vi "cipher data.vi"(8 "error in":errorcluster, 10 "data in":string, 11 "lvlibcrypto digest in":refnum<class "lvlibcrypto cipher.lvclass">) -> (0 "error out":errorcluster, 2 "data out":string, 3 "lvlibcrypto digest out":refnum<class "lvlibcrypto cipher.lvclass">)   [LabVIEW 2016, in "lvlibcrypto cipher.lvclass"]
uses:
  lvlibcrypto cipher.lvclass
  lvlibcrypto cipher.lvclass/lvlibcrypto cipher.ctl
  lv tls dll.lvlib
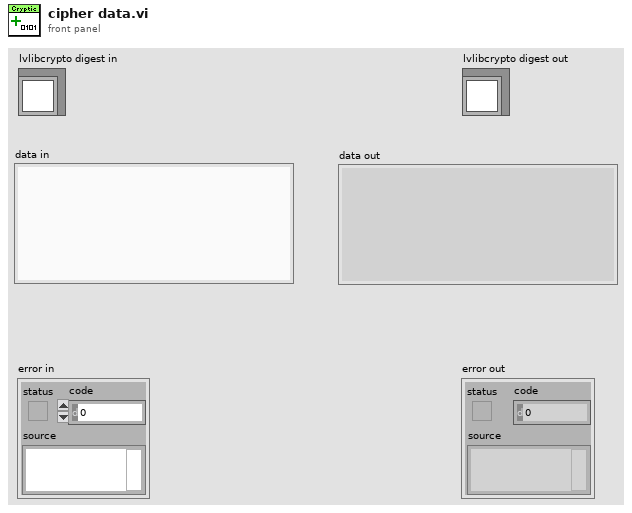
[diagram p1: front panel]
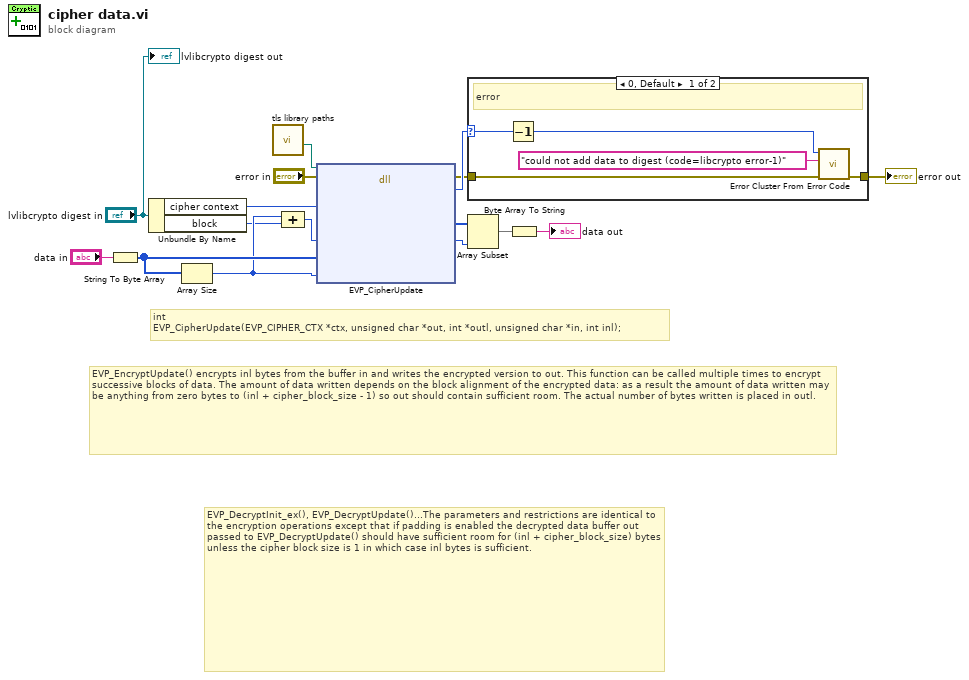
[diagram p0: block diagram]
diagram:
  # "EVP_DecryptInit_ex(), EVP_DecryptUpdate()...The parameters and restrictions are identical to the encryption operations except that if padding is enabled the decrypted data buffer out passed to EVP_DecryptUpdate() should have sufficient room for (inl + cipher_block_size) bytes unless the cipher block size is 1 in which case inl bytes is sufficient."
  # "EVP_EncryptUpdate() encrypts inl bytes from the buffer in and writes the encrypted version to out. This function can be called multiple times to encrypt successive blocks of data. The amount of data written depends on the block alignment of the encrypted data: as a result the amount of data written may be anything from zero bytes to (inl + cipher_block_size - 1) so out should contain sufficient room. The actual number of bytes written is placed in outl."
  # "int \nEVP_CipherUpdate(EVP_CIPHER_CTX *ctx, unsigned char *out, int *outl, unsigned char *in, int inl);"
  n1 = String To Byte Array(string="data in") -> (unsigned byte array=w4:u8[])
  n2 = Unbundle By Name("lvlibcrypto digest in") -> ("cipher context"=w10:u64, "block"=w2:i32)
  n3 = Array Size(array=w4) -> (size(s)=w3:i32)
  n4 = call "tls library paths.vi"() -> ("libcrypto"=w15:path)  [unwired: 8 in, 3 out]
  n5 = Compound Arithmetic op=ADD(w3, w2) -> (w1:i32)
  n6 = dll-call lib="C:/Users/IEUser/Desktop/tlssimple/libcrypto-41.dll" fn="EVP_CipherUpdate"(path in=w15, error in="error in", "context"=w10, "outlength"=w1, "in"=w4, "inlength"=w3) -> (error out=w11:errorcluster, "ret"=w12:i32, "out"=w7:u8[], "outlength"=w5:i32)  [unwired: 5 in, 1 out]
  n7 = case shown="0, Default" w12 {
    selector: w12 -> [w19 _]
    tunnel: [w20 w22] -> w14
    tunnel: w11 -> [w21 w22]
    frame 0, Default {
      # "error"
      n8 = Decrement(x=w19) -> (x-1=w18:i32)
      n9 = call <vilib>:"Error Cluster From Error Code.vi"("error in (no error)"=w21, "error message (\"\")"="could not add data to digest (code=libcrypto error-1)" ("error message (\"\")"), "error code (0)"=w18) -> ("error out"=w20:errorcluster)  [unwired: 6 in]
    }
    frame 1 {
      # "success"
    }
  }
  "error out" <- w14
  n10 = Array Subset(array=w7, length=w5) -> (w6:u8[])  [unwired: 1 in]
  n11 = Byte Array To String(unsigned byte array=w6) -> (string=→"data out":string)
  "lvlibcrypto digest out" <- "lvlibcrypto digest in"
